vi "Do Core.vi"(8 "error in":errorcluster, 9 "Actor in":refnum<class "Actor.lvclass">, 11 "Perform Action on Target Msg":refnum<class "Perform Action on Target Msg.lvclass">) -> (0 "error out":errorcluster, 1 "Actor out":refnum<class "Actor.lvclass">, 2 "Reply":variant)   [LabVIEW 2023, in "IStudy Actor.lvlib" / "Perform Action on Target Msg.lvclass"]
doc: "(<B>Filename</B>: Actor Framework.lvlib:Reply Msg.lvclass:Do Core.vi)\n\nDefines what an actor does when it receives <B>Reply Message</B>. This method also defines the <B>Reply</B> that is returned to the actor that sent <B>Reply Message</B>.\n\nBy default, this method does nothing, and <B>Reply</B> is the ancestor Message class. A child class must override this method to define behavior and specify a child of the Message class to return in the <B>Reply</B> output."
uses:
  Perform Action on Target Msg.lvclass
  <vilib>/ActorFramework/Actor/Actor.lvclass
  IStudy Actor/IStudy Actor.lvclass
  Perform Action on Target Msg.lvclass/Perform Action on Target Msg.ctl
  7c49818c-a8b6-4dc4-b2b0-bd78f06dc2be.vi
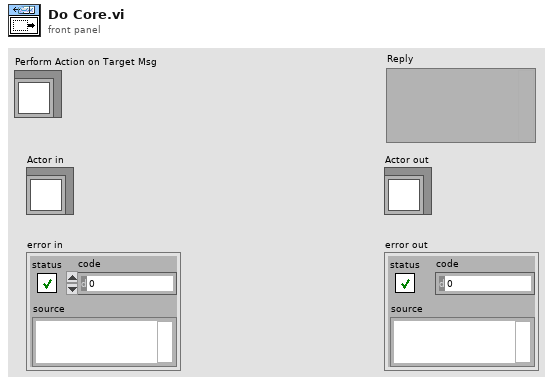
[diagram p1: front panel]
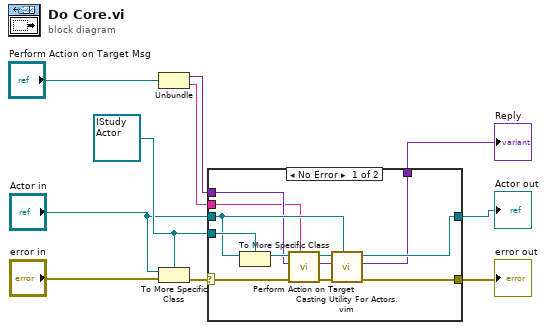
[diagram p0: block diagram]
diagram:
  w8 = refnum<class "IStudy Actor.lvclass"> refnum ("Actor in")
  n1 = Unbundle("Perform Action on Target Msg") -> (w7:variant, w6:string)
  n2 = To More Specific Class(target class=w8, reference="Actor in", error in="error in") -> (error out=w9:errorcluster)  [unwired: 1 out]
  n3 = case shown="No Error" w9 {
    selector: w9 -> [w21 w23]
    tunnel: [w15 w23] -> w2
    tunnel: [w16 w22] -> w3
    tunnel: "Actor in" -> [w18 w22]
    tunnel: w8 -> [w19 _]
    tunnel: w7 -> [w13 _]
    tunnel: w6 -> [w12 _]
    tunnel: [w11 _] -> w1
    frame No Error {
      n4 = To More Specific Class(target class=w19, reference=w18) -> (specific class reference=w20:refnum<class "IStudy Actor.lvclass">)  [unwired: 1 in, 1 out]
      n5 = call-dynamic "Perform Action on Target.vi"("Point dent"=w12, "error in"=w21, "Input"=w13, "IStudy Actor in"=w20) -> ("error out"=w14:errorcluster, "Output"=w11:variant, "IStudy Actor out"=w17:refnum<class "IStudy Actor.lvclass">)  [unwired: 5 in]
      n6 = call "Casting Utility For Actors.vim"("type"=w18, "error in (no error)"=w14, "Actor in"=w17) -> ("error out"=w15:errorcluster, "Actor out"=w16:refnum<class "Actor.lvclass">)  [unwired: 7 in]
    }
    frame Error {
      # "If type check fails, pass the original object out again."
    }
  }
  "error out" <- w2
  "Actor out" <- w3
  "Reply" <- w1
